vi "initiateSubscriberConnection.vi"(3 "topic":string, 4 "Node":string, 5 "URI":string, 6 "Requests In":T1(array[cluster])) -> (0 "error out":errorcluster, 1 "connection ID out":refnum<k5>, 2 "Requests Out":T1(array[cluster]))   [LabVIEW 2010]
panel:
  out "TCP ROS Reply":string
  out "data out":string
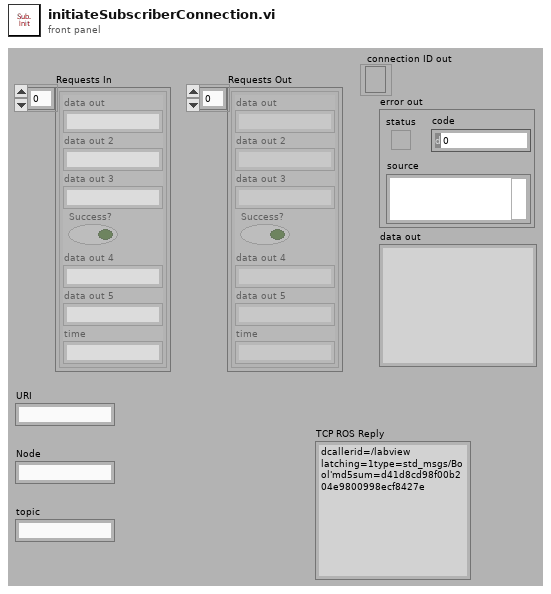
[diagram p1: front panel]
types:
  T1 = cluster{"data out":string, "data out 2":string, "data out 3":string, "Success?":bool, "data out 4":string, "data out 5":string, "time":string}[]
  T2 = cluster{"data out":string, "data out":string, "Node":string, "Success?":bool, "data out 2":string, "data out 3":string}
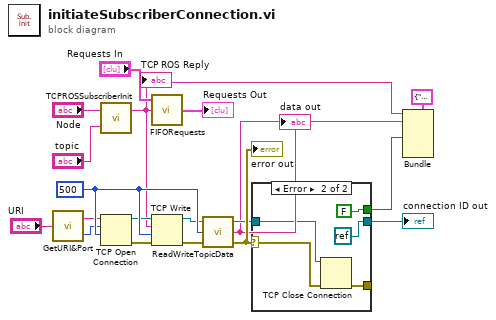
[diagram p0: block diagram]
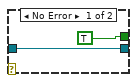
[diagram p2: hidden frame]
diagram:
  w17 = 500 ("timeout ms (60000)")
  n1 = call <userlib>:"GetURI&Port.vi"("URI in"="URI") -> ("Port"=w12:u16, "URI"=w11:string)
  n2 = call <userlib>:"TCPROSSubscriberInit.vi"("topic"="topic", "callerID"="Node") -> ("TCP ROS Reply"=w3:string)  [unwired: 1 out]
  "TCP ROS Reply" <- w3
  n3 = TCP Open Connection(address=w11, remote port or service name=w12, timeout ms (60000)=w17) -> (connection ID=w13:refnum<k5>, error out=w14:errorcluster)  [unwired: 2 in]
  n4 = call <userlib>:"FIFORequests.vi"("data out"=w3, "Requests In"="Requests In") -> ("Requests Out"=→"Requests Out":T1)  [unwired: 1 in]
  n5 = TCP Write(connection ID=w13, data in=w3, error in (no error)=w14, 9:w17) -> (connection ID out=w15:refnum<k5>, error out=w16:errorcluster)  [unwired: 1 out]
  n6 = call <userlib>:"ReadWriteTopicData.vi"("error in (no error)"=w16, "timeout ms (1000)"=w17, "connection ID in"=w15) -> ("error out"=w7:errorcluster, "data out"=w2:string, "connection ID out"=w6:refnum<k5>)
  "error out" <- w7
  "data out" <- w2
  n7 = case shown="Error" w7 {
    selector: w7 -> [_ w23]
    tunnel: [w21 refnum<k0> refnum] -> w5
    tunnel: w6 -> [w21 w24]
    tunnel: [TRUE FALSE] -> w1
    tunnel: [_ w22] -> _
    frame No Error {
    }
    frame Error {
      n8 = TCP Close Connection(connection ID=w24, error in (no error)=w23) -> (error out=w22:errorcluster)  [unwired: 1 in, 1 out]
    }
  }
  "connection ID out" <- w5
  n9 = Bundle(cluster=T2 {"data out"="", "data out"="", "Node"="", "Success?"=FALSE, "data out 2"="", "data out 3"=""} ("New One"), "data out"=w3, "data out"=w2, "Success?"=w1) -> ()  [unwired: 3 in, 1 out]
